vi "Instrument Do Core.vi"(8 "error in (no error)":errorcluster, 9 "Instrument in":refnum<class "Instrument Driver.lvclass">, 10 "Actor in":refnum<class "Actor.lvclass">, 11 "Instrument Msg in":refnum<class "Instrument Msg.lvclass">) -> (0 "error out":errorcluster, 1 "Instrument out":refnum<class "Instrument Driver.lvclass">, 2 "Actor out":refnum<class "Actor.lvclass">, 3 "Instrument Msg out":refnum<class "Instrument Msg.lvclass">, 5 "Data":refnum<class "Data.lvclass">)   [LabVIEW 2020, in "Instrument Handler.lvlib" / "Instrument Msg.lvclass"]
doc: "Message interaction with any instrument is handled by the Instrument Do Core.\n\nThe default implementation does nothing."
uses:
  Instrument Msg.lvclass
  PPL/HDH.Actor Framework.Core.Actor.lvlibp/1abvi3w/vi.lib/ActorFramework/Actor/Actor.lvclass
  PPL/HDH.Data.Generic.lvlibp/Data.lvclass
  PPL/HDH.Actor Framework.Core.Instrument Driver.lvlibp/Instrument Driver/Instrument Driver.lvclass
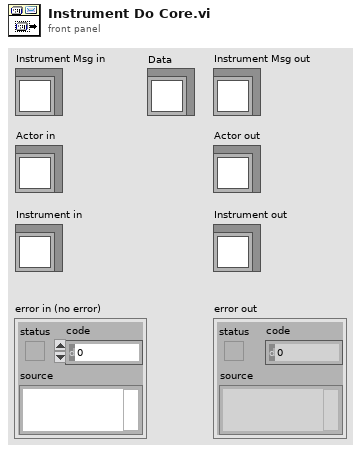
[diagram p1: front panel]
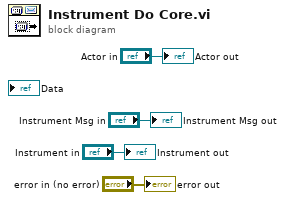
[diagram p0: block diagram]
diagram:
  "error out" <- "error in (no error)"
  "Instrument Msg out" <- "Instrument Msg in"
  "Actor out" <- "Actor in"
  "Instrument out" <- "Instrument in"
